vi "Relative Move DEMO.vi"(8 "error in (no error)":errorcluster, 9 "Axis (1..4)":u16(ring)=1 items=["X"=1, "Y"=2, "Z"=3, "Rotary"=4], 10 "Relative Move, counts":i32, 11 "VISA resource name":refnum<visa-resource-name>) -> (0 "error out":errorcluster, 1 "current position, counts":i32, 3 "VISA resource out":refnum<visa-resource-name>)   [LabVIEW 2017]
panel:
  out "Limit Switch Activated":bool
  out "Positions, counts":i32[](array[numeric])
  in  "stop":bool
  out "i":i32
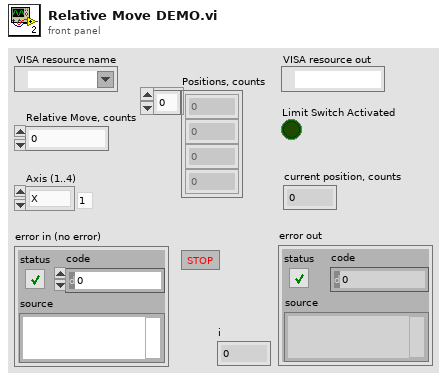
[diagram p1: front panel]
types:
  T1 = enum16{"Cmd-Response", "Write Only", "Read Only"}
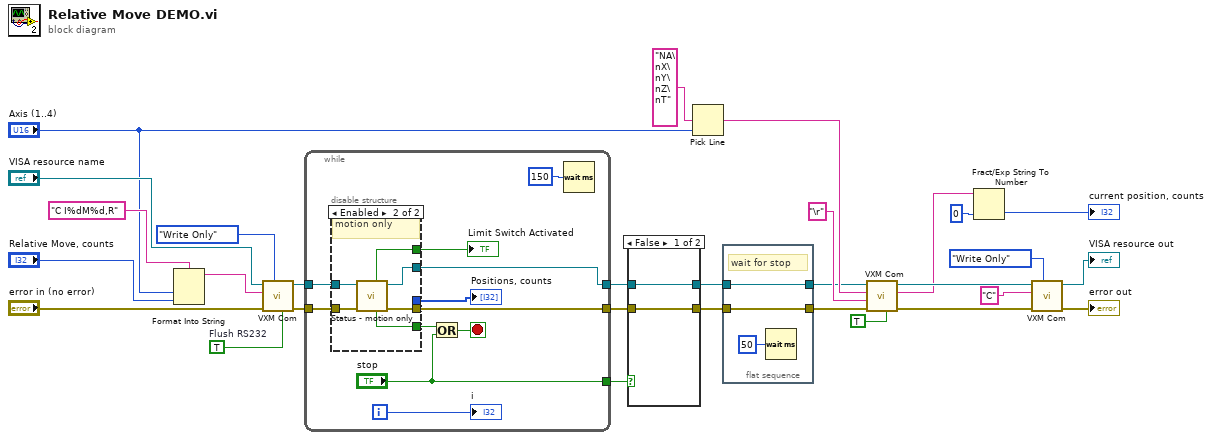
[diagram p0: block diagram]
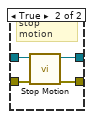
[diagram p2: hidden frame]
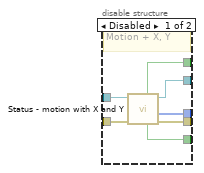
[diagram p3: hidden frame]
diagram:
  w2 = TRUE  # Flush RS232
  n1 = Format Into String(format string="C I%dM%d,R", "Axis (1..4)", "Relative Move, counts") -> (resulting string=w27:string)  [unwired: 2 in, 1 out]
  n2 = call "VXM Com.vi"("Flush RS232"=w2, "Operation"=T1."Write Only", "error in (no error)"="error in (no error)", "Write Buffer ('/' codes)"=w27, "VISA resource name"="VISA resource name") -> ("error out"=w11:errorcluster, "VISA resource out"=w10:refnum<visa-resource-name>)  [unwired: 4 in, 1 out]
  n3 = while {
    tunnel: w11 -> [w37]
    tunnel: [w36] -> w9
    tunnel: ["stop"] -> w7
    tunnel: w10 -> [w33]
    tunnel: [w32] -> w8
    i -> [w40]
    stop <- w41 stop-if-true
    n4 = disable-structure shown="Enabled" {
      disable-tunnel: w37 -> [w48 w53]
      disable-tunnel: [w47 w51] -> w36
      disable-tunnel: [w46 _] -> w35
      disable-tunnel: [w45 w50] -> w34
      disable-tunnel: w33 -> [w44 w54]
      disable-tunnel: [w43 w52] -> w32
      disable-tunnel: [w42 w49] -> w31
      frame Disabled {
        # "Motion + X, Y"
        n5 = call "Status - motion with X and Y.vi"("error in (no error)"=w48, "VISA resource name"=w44) -> ("error out"=w47:errorcluster, "Positions, counts"=w46:i32[], "VISA resource out"=w43:refnum<visa-resource-name>, "Motion Stopped"=w45:bool, "Limit Switch Activated"=w42:bool)  [unwired: 5 in]
      }
      frame Enabled {
        # "motion only"
        n6 = call "Status - motion only.vi"("error in (no error)"=w53, "VISA resource name"=w54) -> ("error out"=w51:errorcluster, "VISA resource out"=w52:refnum<visa-resource-name>, "Motion Stopped"=w50:bool, "Limit Switch Activated"=w49:bool)  [unwired: 6 in]
      }
    }
    "Positions, counts" <- w35
    "Limit Switch Activated" <- w31
    n7 = Or(x=w34, y="stop") -> (x .or. y?=w41:bool)
    n8 = Wait (ms)(milliseconds to wait=u32 150) -> ()  [unwired: 1 out]
    "i" <- w40
  }
  n9 = case shown="False" w7 {
    tunnel: w9 -> [w56 w60]
    tunnel: [w56 w59] -> w4
    tunnel: w8 -> [w55 w58]
    tunnel: [w55 w57] -> w6
    frame False {
    }
    frame True {
      # "stop motion"
      n10 = call "Stop Motion.vi"("error in (no error)"=w60, "VISA resource name"=w58) -> ("error out"=w59:errorcluster, "VISA resource out"=w57:refnum<visa-resource-name>)  [unwired: 8 in]
    }
  }
  n11 = Pick Line(multi-line string="NA\nX\nY\nZ\nT", line index="Axis (1..4)") -> (output string=w17:string)  [unwired: 1 in]
  n12 = flat-sequence {
    tunnel: [w63] -> w5
    tunnel: w6 -> [w63]
    tunnel: [w62] -> w3
    tunnel: w4 -> [w62]
    frame #0 {
      # "wait for stop"
      n13 = Wait (ms)(milliseconds to wait=u32 50) -> ()  [unwired: 1 out]
    }
  }
  n14 = call "VXM Com.vi"("Flush RS232"=TRUE, "error in (no error)"=w3, "Termination String ('/' codes)"="\r", "Write Buffer ('/' codes)"=w17, "VISA resource name"=w5) -> ("error out"=w24:errorcluster, "Response String ('/' codes)"=w21:string, "VISA resource out"=w23:refnum<visa-resource-name>)  [unwired: 4 in]
  n15 = Fract/Exp String To Number(string=w21, default (0 dbl)=0 ("default (0 DBL)")) -> (number=→"current position, counts":i32)  [unwired: 2 in, 1 out]
  n16 = call "VXM Com.vi"("Operation"=T1."Write Only", "error in (no error)"=w24, "Write Buffer ('/' codes)"="C" ("Write Buffer"), "VISA resource name"=w23) -> ("error out"=→"error out":errorcluster, "VISA resource out"=→"VISA resource out":refnum<visa-resource-name>)  [unwired: 5 in, 1 out]
